vi "Helper - ManualRudder.vi"(4 "Array":dbl[](array[numeric]), 5 "Straight":bool, 6 "Full Starboard":bool, 7 "Starboard":bool, 8 "Port":bool, 9 "Full Port":bool) -> (2 "Array 2":dbl[](array[numeric]))   [LabVIEW 2011]
panel:
  # "This control is passed an array"
  # "This indicator shows the output"
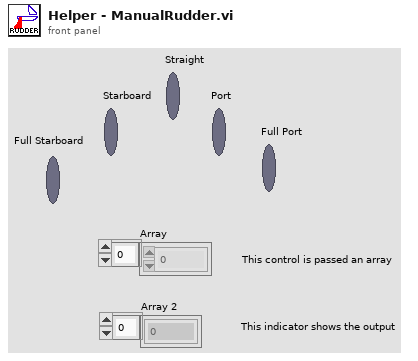
[diagram p1: front panel]
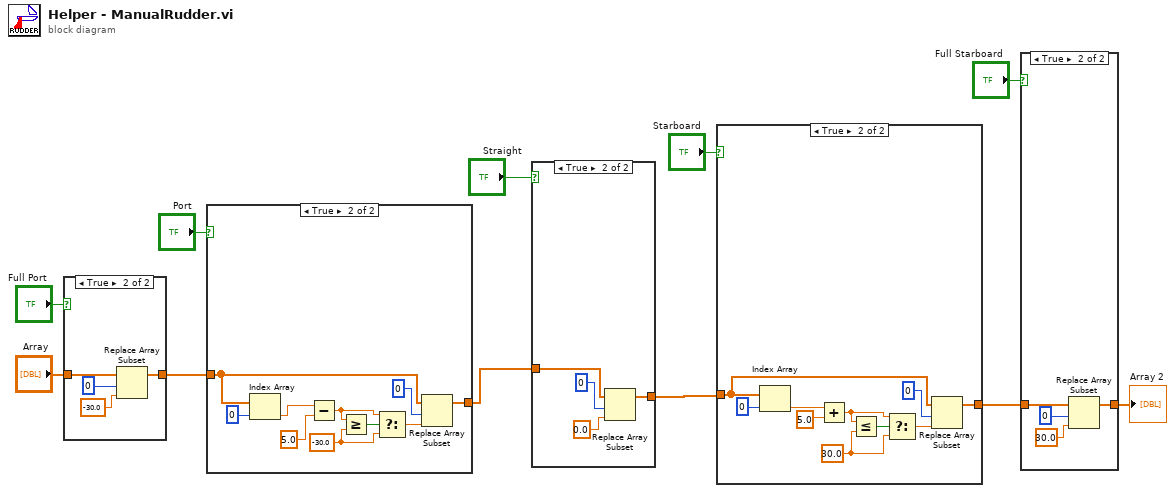
[diagram p0: block diagram]
diagram:
  n1 = case shown="True" "Full Port" {
    tunnel: "Array" -> [w12 w14]
    tunnel: [w12 w16] -> w9
    frame False {
    }
    frame True {
      n2 = Replace Array Subset(array=w14, new element=-30.0 ("new element/subarray"), index=0) -> (w16:dbl[])
    }
  }
  n3 = case shown="True" "Port" {
    tunnel: w9 -> [w17 w26]
    tunnel: [w17 w27] -> w2
    frame False {
    }
    frame True {
      w20 = -30.0
      n4 = Index Array(array=w26, index=0) -> (element=w19:dbl)
      n5 = Subtract(x=w19, y=5.0) -> (x-y=w22:dbl)
      n6 = Greater Or Equal?(x=w22, y=w20) -> (x >= y?=w23:bool)
      n7 = Select(t=w22, s=w23, f=w20) -> (s? t:f=w21:dbl)
      n8 = Replace Array Subset(array=w26, new element=w21, index=0) -> (w27:dbl[])
    }
  }
  n9 = case shown="True" "Straight" {
    tunnel: w2 -> [w28 w31]
    tunnel: [w28 w32] -> w1
    frame False {
    }
    frame True {
      n10 = Replace Array Subset(array=w31, new element=0.0 ("new element/subarray"), index=0) -> (w32:dbl[])
    }
  }
  n11 = case shown="True" "Starboard" {
    tunnel: w1 -> [w33 w42]
    tunnel: [w33 w43] -> w6
    frame False {
    }
    frame True {
      w37 = 30.0
      n12 = Index Array(array=w42, index=0) -> (element=w34:dbl)
      n13 = Add(x=w34, y=5.0 ("x")) -> (x+y=w35:dbl)
      n14 = Less Or Equal?(x=w35, y=w37) -> (x <= y?=w38:bool)
      n15 = Select(t=w35, s=w38, f=w37) -> (s? t:f=w39:dbl)
      n16 = Replace Array Subset(array=w42, new element=w39, index=0) -> (w43:dbl[])
    }
  }
  n17 = case shown="True" "Full Starboard" {
    tunnel: w6 -> [w44 w48]
    tunnel: [w44 w46] -> w5
    frame False {
    }
    frame True {
      n18 = Replace Array Subset(array=w48, new element=30.0 ("new element/subarray"), index=0) -> (w46:dbl[])
    }
  }
  "Array 2" <- w5
